vi "fix close.vi"(8 "error in":errorcluster, 11 "vi in":refnum<vi>) -> (0 "error out":errorcluster)   [LabVIEW 2013, in "DecideModuleFeatures.lvclass"]
uses:
  DecideModuleFeatures.lvclass
  <vilib>/Utility/traverseref.llb/TRef TravTarget.ctl
  <vilib>/Utility/traverseref.llb/VI Scripting - Traverse.lvlib
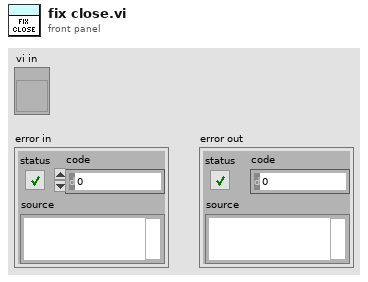
[diagram p1: front panel]
types:
  T1 = typedef "TRef TravTarget.ctl" = enum16{"FP", "BD", "Other"}
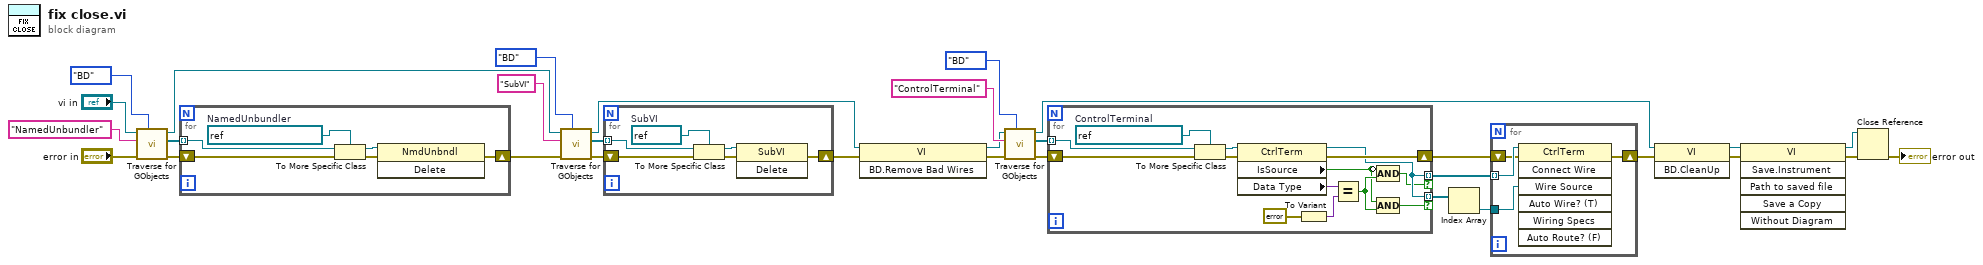
[diagram p0: block diagram]
diagram:
  n1 = call <vilib>:"Traverse for GObjects.vi"("Traverse Target"=TRef_TravTarget."BD", "error in (no error)"="error in", "Class Name"="NamedUnbundler", "VI Refnum"="vi in") -> ("error out"=w27:errorcluster, "References"=w28:refnum<vi>[], "dup VI Refnum"=w21:refnum<vi>)  [unwired: 4 in, 1 out]
  n2 = for {
    tunnel: w28 -> [w36] mode=indexing
    shift-right: [w32] -> w20
    shift-left: w27 -> [w35]
    w37 = refnum<vi> refnum  # NamedUnbundler
    n3 = To More Specific Class(target class=w37, reference=w36, error in=w35) -> (specific class reference=w34:refnum<vi>, error out=w33:errorcluster)
    n4 = invoke class="NmdUnbndl" method="Delete"(reference=w34, error in=w33) -> (error out=w32:errorcluster)  [unwired: 1 in, 2 out]
  }
  n5 = call <vilib>:"Traverse for GObjects.vi"("Traverse Target"=TRef_TravTarget."BD", "error in (no error)"=w20, "Class Name"="SubVI", "VI Refnum"=w21) -> ("error out"=w24:errorcluster, "References"=w23:refnum<vi>[], "dup VI Refnum"=w13:refnum<vi>)  [unwired: 4 in, 1 out]
  n6 = for {
    tunnel: w23 -> [w42] mode=indexing
    shift-right: [w38] -> w15
    shift-left: w24 -> [w41]
    w43 = refnum<vi> refnum  # SubVI
    n7 = To More Specific Class(target class=w43, reference=w42, error in=w41) -> (specific class reference=w40:refnum<vi>, error out=w39:errorcluster)
    n8 = invoke class="SubVI" method="Delete"(reference=w40, error in=w39) -> (error out=w38:errorcluster)  [unwired: 1 in, 2 out]
  }
  n9 = invoke class="VI" method="BD.Remove Bad Wires"(reference=w13, error in=w15) -> (reference out=w12:refnum<vi>, error out=w14:errorcluster)  [unwired: 1 in, 1 out]
  n10 = call <vilib>:"Traverse for GObjects.vi"("Traverse Target"=TRef_TravTarget."BD", "error in (no error)"=w14, "Class Name"="ControlTerminal", "VI Refnum"=w12) -> ("error out"=w17:errorcluster, "References"=w18:refnum<vi>[], "dup VI Refnum"=w10:refnum<vi>)  [unwired: 4 in, 1 out]
  n11 = for {
    tunnel: w18 -> [w56] mode=indexing
    shift-right: [w49] -> w5
    shift-left: w17 -> [w55]
    tunnel: [w48] -> w7 mode=indexing if=w47
    tunnel: [w48] -> w8 mode=indexing if=w44
    w57 = refnum<vi> refnum  # ControlTerminal
    n12 = To More Specific Class(target class=w57, reference=w56, error in=w55) -> (specific class reference=w54:refnum<vi>, error out=w53:errorcluster)
    n13 = property class="CtrlTerm"(reference=w54, error in=w53) -> (reference out=w48:refnum<vi>, error out=w49:errorcluster, "IsSource"=w45:bool, "Data Type"=w52:variant)
    n14 = To Variant(anything=errorcluster {"status"=FALSE, "code"=0, "source"=""} ("error out")) -> (Variant=w50:variant)
    n15 = Equal?(x=w52, y=w50) -> (x = y?=w46:bool)
    n16 = Compound Arithmetic op=AND(invert w45, w46) -> (w44:bool)
    n17 = Compound Arithmetic op=AND(w45, w46) -> (w47:bool)
  }
  n18 = Index Array(array=w7) -> (element=w6:refnum<vi>)  [unwired: 1 in]
  n19 = for {
    tunnel: w8 -> [w61] mode=indexing
    tunnel: w6 -> [w60]
    shift-right: [w58] -> w4
    shift-left: w5 -> [w59]
    n20 = invoke class="CtrlTerm" method="Connect Wire"(reference=w61, error in=w59, "Wire Source"=w60) -> (error out=w58:errorcluster)  [unwired: 4 in, 6 out]
  }
  n21 = invoke class="VI" method="BD.CleanUp"(reference=w10, error in=w4) -> (reference out=w9:refnum<vi>, error out=w11:errorcluster)  [unwired: 1 in, 1 out]
  n22 = invoke class="VI" method="Save.Instrument"(reference=w9, error in=w11) -> (reference out=w30:refnum<vi>, error out=w31:errorcluster)  [unwired: 4 in, 4 out]
  n23 = Close Reference(reference=w30, error in (no error)=w31) -> (error out=→"error out":errorcluster)
